vi "Initialize UI Elements.vi"(8 "error in":errorcluster, 10 "References":refnum<vi>[](array[refnum]), 11 "NumSlots":i32) -> (0 "error out":errorcluster, 1 "Programming Mode Out":T1[](array[typedef]))   [LabVIEW 2019, in "SEECD System Explorer.lvlib"]
doc: "Initialize Slot Programming Modes Controls (8 elements). We use individual elements because we want to be able to control respective \"Enable State\"."
uses:
  SEECD System Explorer.lvlib
  Type Defs/Slot Programming Mode.ctl
  Type Defs/Slot - Configuration.ctl
panel:
  in  "Slot Programming Mode":T1=enum."Scan Engine"
  in  "Slot 2":string
  in  "Slot":T2={"Slot"="", "Module Name"="", "Slot Programming Mode"=enum."Scan Engine"}
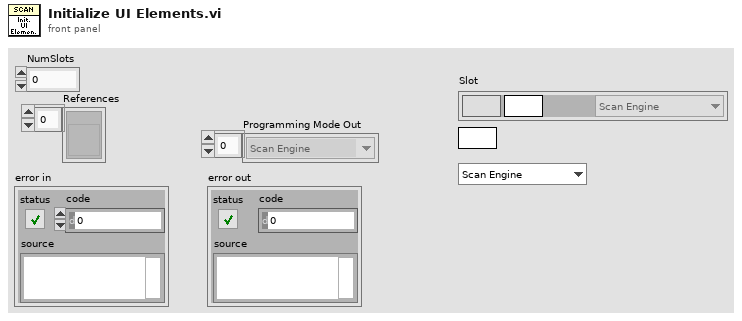
[diagram p1: front panel]
types:
  T1 = typedef "SEECD System Explorer.lvlib/Slot Programming Mode.ctl" = enum16{"Don't Modify", "Scan Engine", "LabVIEW FPGA", "NI-DAQmx"}
  T2 = typedef "SEECD System Explorer.lvlib/Slot - Configuration.ctl" = cluster{"Slot":string, "Module Name":string, "Slot Programming Mode":T1}
  T3 = enum8{"Enabled", "Disabled", "Disabled and Grayed Out"}
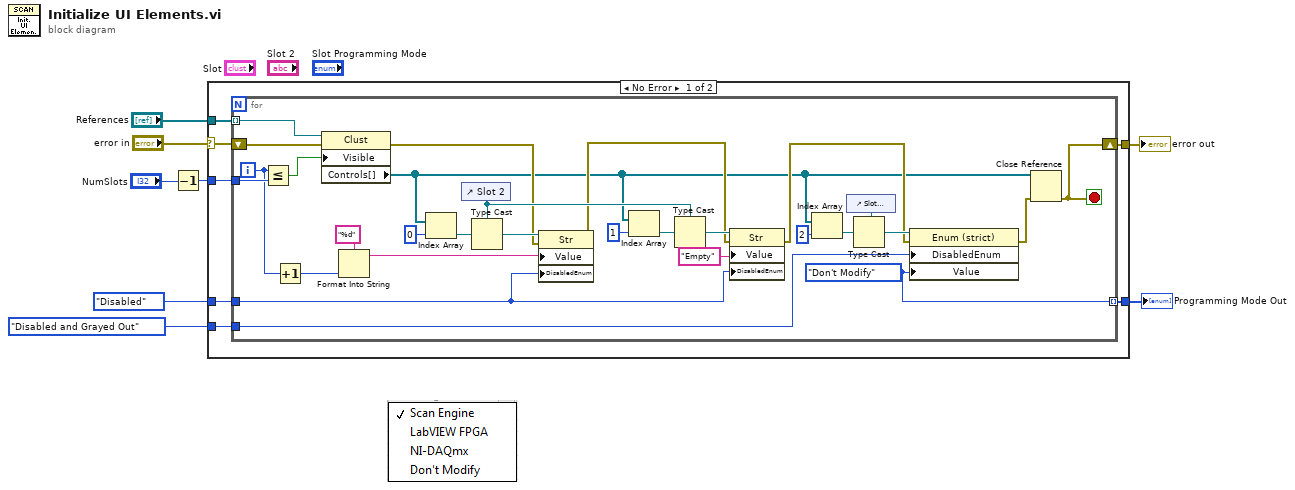
[diagram p0: block diagram]
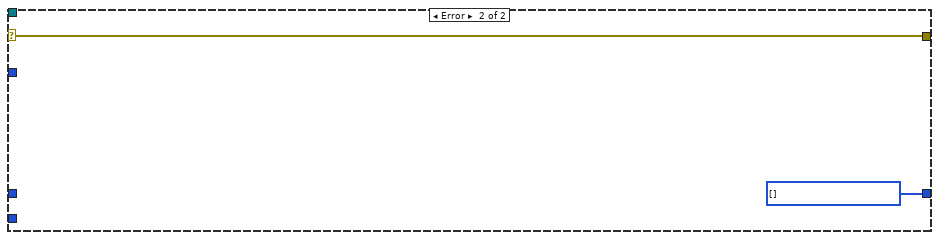
[diagram p2: hidden frame]
diagram:
  n1 = Decrement(x="NumSlots") -> (x-1=w4:i32)
  n2 = case shown="No Error" "error in" {
    selector: "error in" -> [w12 w46]
    tunnel: "References" -> [w15 _]
    tunnel: T3."Disabled" ("Disabled") -> [w14 _]
    tunnel: [w13 w46] -> w7
    tunnel: w4 -> [w11 _]
    tunnel: T3."Disabled and Grayed Out" ("Disabled") -> [w10 _]
    tunnel: [w9 w45] -> w2
    frame No Error {
      n3 = for {
        tunnel: w15 -> [w43] mode=indexing
        shift-right: [w18] -> w13
        shift-left: w12 -> [w42]
        tunnel: w14 -> [w29]
        tunnel: w11 -> [w44]
        tunnel: w10 -> [w24]
        tunnel: [w23] -> w9 mode=indexing
        i -> [w38]
        stop <- w18 stop-if-true
        w23 = Slot_Programming_Mode."Don't Modify" ("Value")
        n4 = Less Or Equal?(x=w38, y=w44) -> (x <= y?=w16:bool)
        n5 = Increment(x=w38) -> (x+1=w37:i32)
        n6 = property class="Clust"(reference=w43, error in=w42, "Visible"=w16) -> (error out=w22:errorcluster, "Controls[]"=w17:refnum<vi>[])  [unwired: 1 out]
        n7 = Format Into String(format string="%d", w37) -> (resulting string=w35:string)  [unwired: 2 in, 1 out]
        n8 = Index Array(array=w17, index=0) -> (element=w40:refnum<vi>)
        n9 = control-ref of="Slot 2"() -> (w31:refnum<vi>)
        n10 = Type Cast(type=w31, x=w40) -> (*(type *) &x=w39:refnum<vi>)
        n11 = property class="Str"(reference=w39, error in=w22, "Value"=w35, "DisabledEnum"=w29) -> (error out=w21:errorcluster)  [unwired: 1 out]
        n12 = Index Array(array=w17, index=1) -> (element=w33:refnum<vi>)
        n13 = Type Cast(type=w31, x=w33) -> (*(type *) &x=w34:refnum<vi>)
        n14 = property class="Str"(reference=w34, error in=w21, "Value"="Empty", "DisabledEnum"=w29) -> (error out=w19:errorcluster)  [unwired: 1 out]
        n15 = Index Array(array=w17, index=2) -> (element=w26:refnum<vi>)
        n16 = control-ref of="Slot Programming Mode"() -> (w27:refnum<vi>)
        n17 = Type Cast(type=w27, x=w26) -> (*(type *) &x=w25:refnum<vi>)
        n18 = property class="Enum (strict)"(reference=w25, error in=w19, "DisabledEnum"=w24, "Value"=w23) -> (error out=w20:errorcluster)  [unwired: 1 out]
        n19 = Close Reference(reference=w17, error in (no error)=w20) -> (error out=w18:errorcluster)
      }
    }
    frame Error {
      w45 = T1[] [] items=["Don't Modify", "Scan Engine", "LabVIEW FPGA", "NI-DAQmx"]
    }
  }
  "error out" <- w7
  "Programming Mode Out" <- w2
